vi "Auto Near Switch.vi"(9 "Time to wait (min 50ms)":dbl=50.0, 10 "Right?":bool) -> ()   [LabVIEW 2017]
uses:
  Auto switch direita.ctl
  LabVIEW_is_Under_Control.lib/Util/Unpack Gamepad/Button Cluster.ctl
  Team Code/Robot Global Data.vi
panel:
  in  "90_time_limit":dbl=1800.0
  in  "Time_limit_fwd_2":dbl=1500.0 format="%#_13g"
  in  "Time_Limit_fwd":dbl=4000.0 format="%#_13g"
  in  "Delay fwd 2":i32=10
  in  "DistanceAfterTurn":dbl=40.0
  in  "Delay Turn":i32=150
  in  "Turn":dbl=-90.0 format="%#_13g"
  in  "Delay Fwd":i32=100
  in  "DistanceSwitch":dbl=380.0
  out "auto state":T1=enum."Girando"
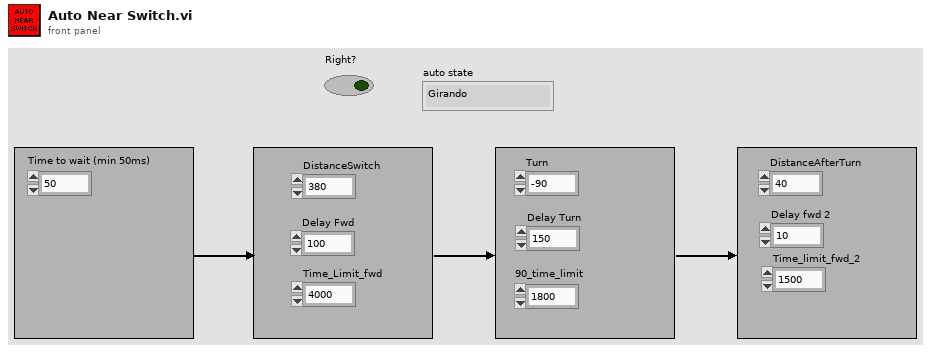
[diagram p1: front panel]
types:
  T1 = typedef "Auto switch direita.ctl" = enum16{"Zerandosensor", "Girando", "Andando", "Jogando", "Andando2", "Finalizando", "Zerandosensor2"}
  T2 = typedef "Button Cluster.ctl" = cluster{"Buttons[0]":bool, "Buttons[1]":bool, "Buttons[2]":bool, "Buttons[3]":bool, "Buttons[4]":bool, "Buttons[5]":bool, "Buttons[6]":bool, "Buttons[7]":bool, "Buttons[8]":bool, "Buttons[9]":bool}
  T3 = cluster{"proportional gain (Kc)":dbl, "integral time (Ti, min)":dbl, "derivative time (Td, min)":dbl}
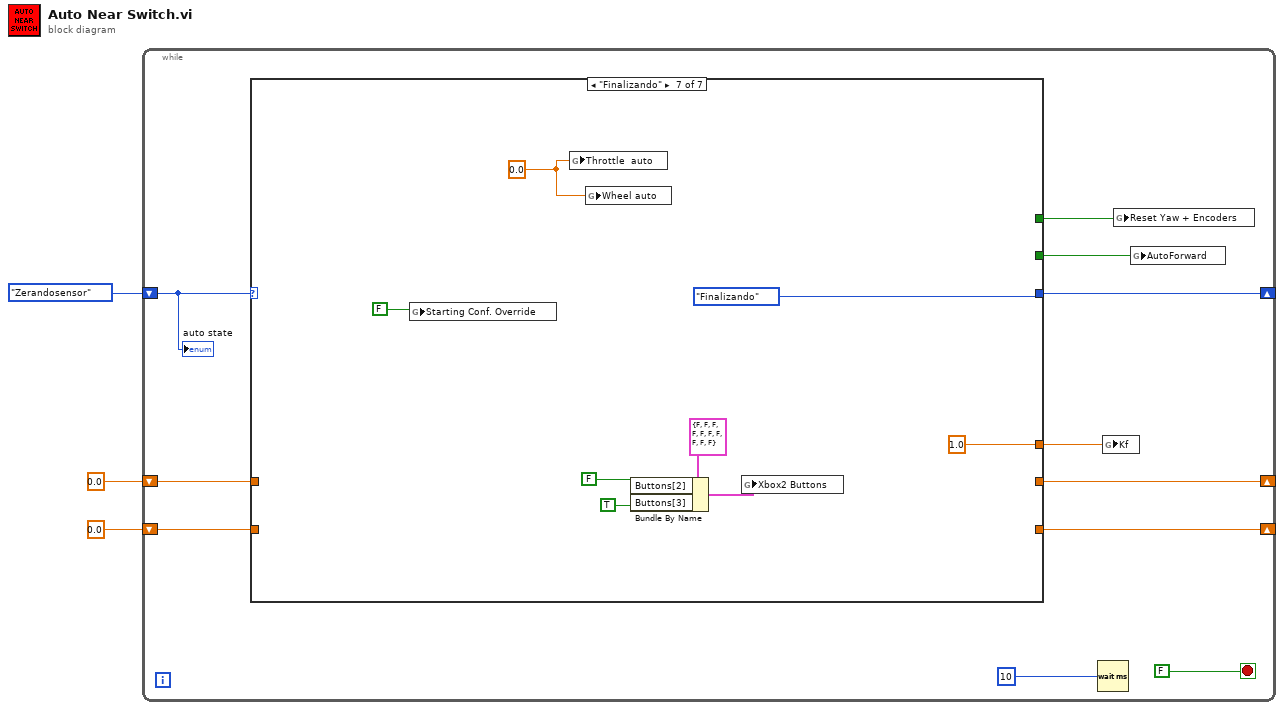
[diagram p0: block diagram]
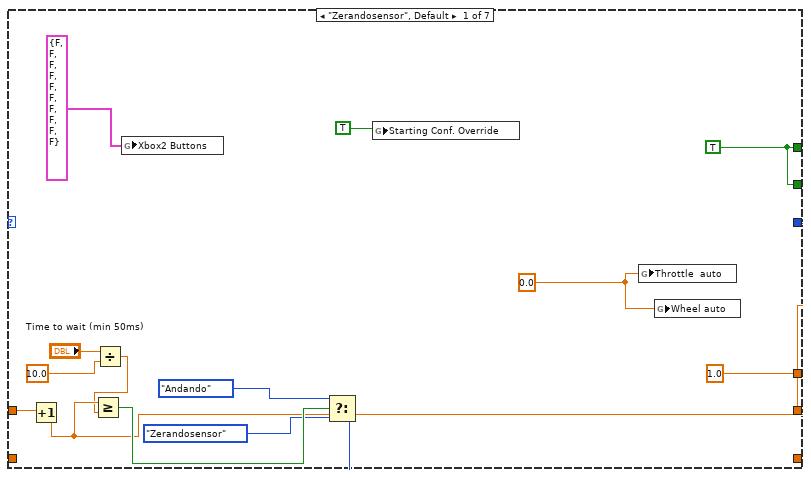
[diagram p2: hidden frame]
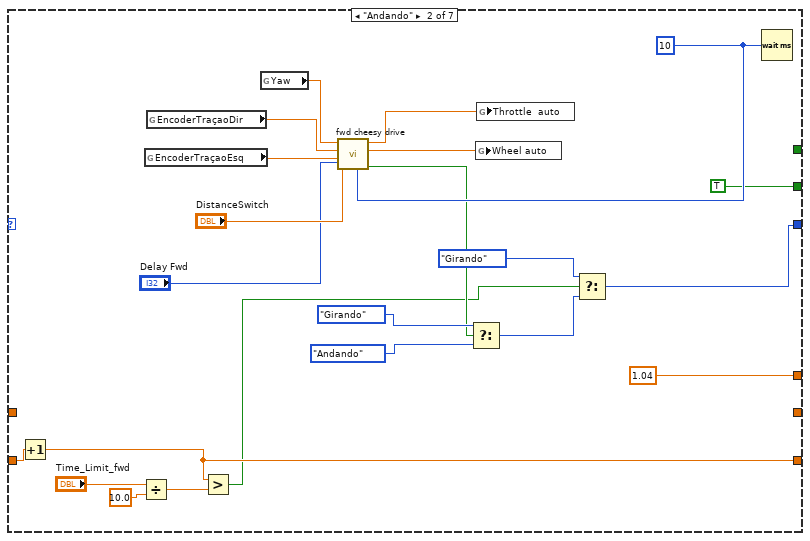
[diagram p3: hidden frame]
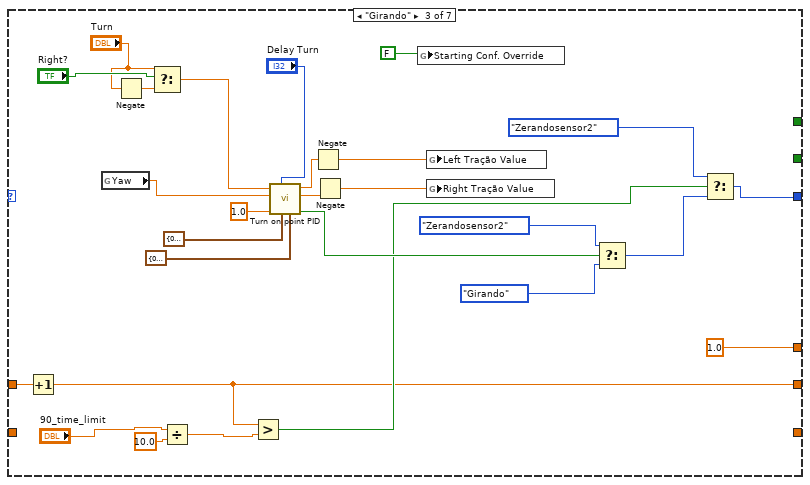
[diagram p4: hidden frame]
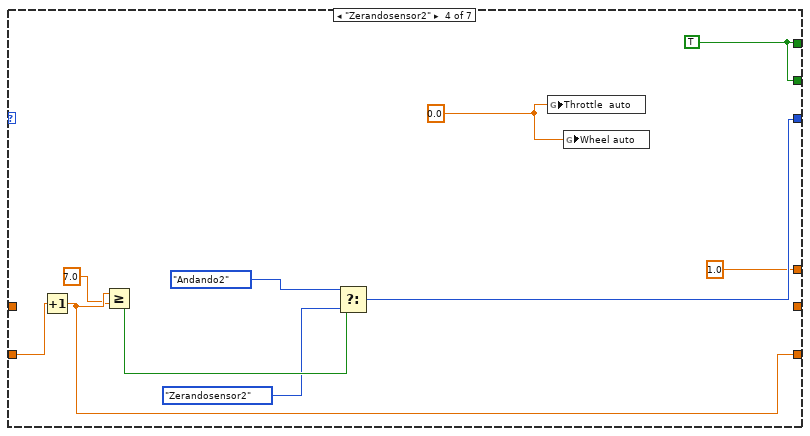
[diagram p5: hidden frame]
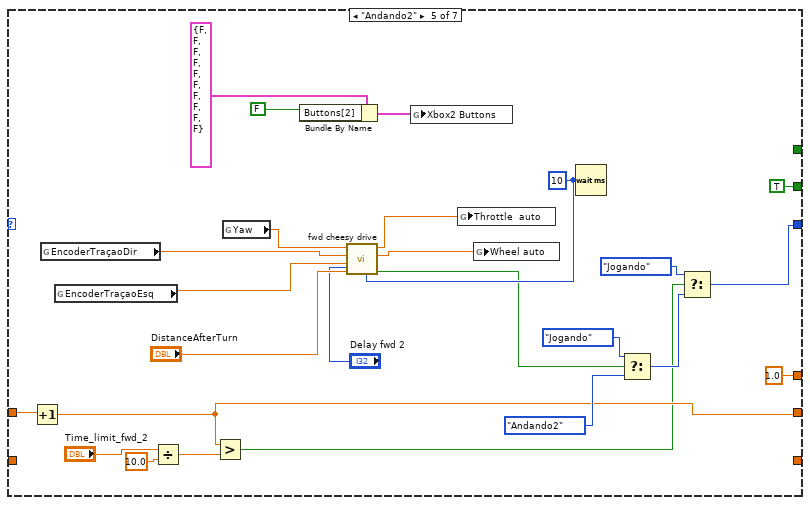
[diagram p6: hidden frame]
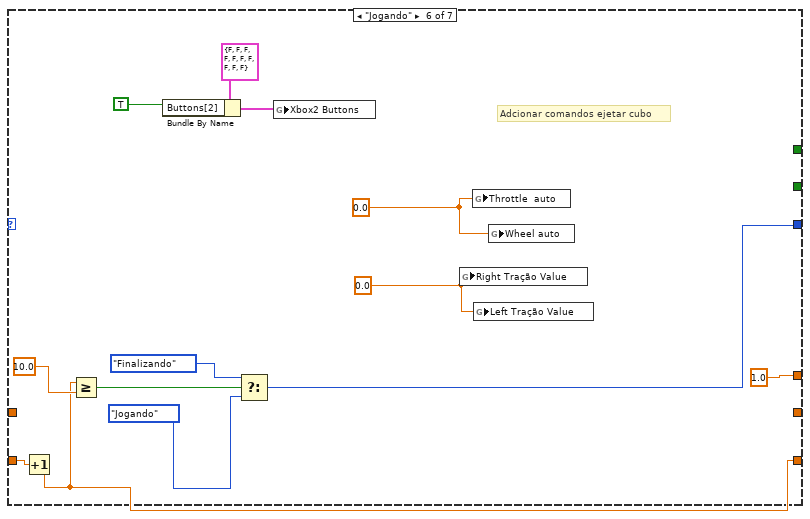
[diagram p7: hidden frame]
diagram:
  n1 = while {
    shift-right: [w10] -> _
    shift-left: Auto_switch_direita."Zerandosensor" -> [w8]
    shift-right: [w11] -> _
    shift-left: 0.0 -> [w12]
    shift-right: [w4] -> _
    shift-left: 0.0 -> [w5]
    stop <- FALSE stop-if-true
    n2 = case shown="\"Finalizando\"" w8 {
      tunnel: w12 -> [w19 _ w55 _ w98 _ _]
      tunnel: [w16 _ w54 _ w97 _ _] -> w11
      tunnel: [w27 w36 w57 w82 w93 w124 Auto_switch_direita."Finalizando"] -> w10
      tunnel: [w24 _ _ w86 _ _ _] -> w7
      tunnel: [w24 TRUE _ w86 TRUE _ _] -> w9
      tunnel: [1.0 1.04 1.0 1.0 1.0 1.0 1.0] -> w6
      tunnel: w5 -> [_ w32 _ w80 _ w120 _]
      tunnel: [_ w31 _ w79 _ w113 _] -> w4
      frame "Zerandosensor", Default {
        w23 = 0.0
        w24 = TRUE
        n3 = Increment(x=w19) -> (x+1=w16:dbl)
        n4 = Divide(x="Time to wait (min 50ms)", y=10.0) -> (x/y=w15:dbl)
        n5 = Greater Or Equal?(x=w16, y=w15) -> (x >= y?=w28:bool)
        n6 = global write "Robot Global Data.vi" "Xbox2 Buttons"(T2 {"Buttons[0]"=FALSE, "Buttons[1]"=FALSE, "Buttons[2]"=FALSE, "Buttons[3]"=FALSE, "Buttons[4]"=FALSE, "Buttons[5]"=FALSE, "Buttons[6]"=FALSE, "Buttons[7]"=FALSE, "Buttons[8]"=FALSE, "Buttons[9]"=FALSE} ("Madcatz Buttons")) -> ()
        n7 = Select(t=Auto_switch_direita."Andando", s=w28, f=Auto_switch_direita."Zerandosensor") -> (s? t:f=w27:T1)
        n8 = global write "Robot Global Data.vi" "Starting Conf. Override"(TRUE) -> ()
        n9 = global write "Robot Global Data.vi" "Throttle  auto"(w23) -> ()
        n10 = global write "Robot Global Data.vi" "Wheel auto"(w23) -> ()
      }
      frame "Andando" {
        w46 = u32 10 ("milliseconds to wait")
        n11 = Increment(x=w32) -> (x+1=w31:dbl)
        n12 = Divide(x="Time_Limit_fwd", y=10.0) -> (x/y=w33:dbl)
        n13 = global read "Robot Global Data.vi" "EncoderTraçaoEsq"() -> (w49:dbl)
        n14 = global read "Robot Global Data.vi" "EncoderTraçaoDir"() -> (w48:dbl)
        n15 = Greater?(x=w31, y=w33) -> (0:w29:bool)
        n16 = global read "Robot Global Data.vi" "Yaw"() -> (w50:dbl)
        n17 = call "fwd cheesy drive.vi"("Loop Timer"=w46, "Time to stop"="Delay Fwd", "Distance"="DistanceSwitch", "Encoder Left"=w49, "Encoder Right"=w48, "Yaw"=w50) -> ("Finished distance"=w30:bool, "Direction"=w44:dbl, "Trottle"=w43:dbl)  [unwired: 2 in, 1 out]
        n18 = Select(t=Auto_switch_direita."Girando", s=w30, f=Auto_switch_direita."Andando") -> (s? t:f=w37:T1)
        n19 = global write "Robot Global Data.vi" "Wheel auto"(w44) -> ()
        n20 = global write "Robot Global Data.vi" "Throttle  auto"(w43) -> ()
        n21 = Select(t=Auto_switch_direita."Girando", s=w29, f=w37) -> (s? t:f=w36:T1)
        n22 = Wait (ms)(milliseconds to wait=w46) -> ()  [unwired: 1 out]
      }
      frame "Girando" {
        n23 = Increment(x=w55) -> (x+1=w54:dbl)
        n24 = global read "Robot Global Data.vi" "Yaw"() -> (w70:dbl)
        n25 = Negate(x="Turn") -> (-x=w65:dbl)
        n26 = Select(t="Turn", s="Right?", f=w65) -> (s? t:f=w63:dbl)
        n27 = Divide(x="90_time_limit", y=10.0) -> (x/y=w61:dbl)
        n28 = Greater?(x=w54, y=w61) -> (0:w59:bool)
        n29 = call "Turn on point PID.vi"("Range"=cluster{"output high":dbl, "output low":dbl} {"output high"=0.65, "output low"=-0.65}, "Gains"=T3 {"proportional gain (Kc)"=0.015, "integral time (Ti, min)"=0.01, "derivative time (Td, min)"=0.0}, "Time to stop"="Delay Turn", "Precision"=1.0, "Yaw"=w70, "Setpoint(degrees)"=w63) -> ("Finished?"=w76:bool, "PWM right"=w72:dbl, "PWM left"=w73:dbl)  [unwired: 3 in]
        n30 = Negate(x=w73) -> (-x=w69:dbl)
        n31 = Negate(x=w72) -> (-x=w68:dbl)
        n32 = global write "Robot Global Data.vi" "Starting Conf. Override"(FALSE) -> ()
        n33 = global write "Robot Global Data.vi" "Left Tração Value"(w69) -> ()
        n34 = global write "Robot Global Data.vi" "Right Tração Value"(w68) -> ()
        n35 = Select(t=Auto_switch_direita."Zerandosensor2", s=w76, f=Auto_switch_direita."Girando") -> (s? t:f=w58:T1)
        n36 = Select(t=Auto_switch_direita."Zerandosensor2", s=w59, f=w58) -> (s? t:f=w57:T1)
      }
      frame "Zerandosensor2" {
        w86 = TRUE
        w87 = 0.0
        n37 = Increment(x=w80) -> (x+1=w79:dbl)
        n38 = Greater Or Equal?(x=w79, y=7.0) -> (x >= y?=w85:bool)
        n39 = Select(t=Auto_switch_direita."Andando2", s=w85, f=Auto_switch_direita."Zerandosensor2") -> (s? t:f=w82:T1)
        n40 = global write "Robot Global Data.vi" "Throttle  auto"(w87) -> ()
        n41 = global write "Robot Global Data.vi" "Wheel auto"(w87) -> ()
      }
      frame "Andando2" {
        w109 = u32 10 ("milliseconds to wait")
        n42 = Increment(x=w98) -> (x+1=w97:dbl)
        n43 = global read "Robot Global Data.vi" "EncoderTraçaoDir"() -> (w91:dbl)
        n44 = global read "Robot Global Data.vi" "EncoderTraçaoEsq"() -> (w111:dbl)
        n45 = Divide(x="Time_limit_fwd_2", y=10.0) -> (x/y=w99:dbl)
        n46 = Greater?(x=w97, y=w99) -> (0:w95:bool)
        n47 = global read "Robot Global Data.vi" "Yaw"() -> (w112:dbl)
        n48 = Bundle By Name(cluster=T2 {"Buttons[0]"=FALSE, "Buttons[1]"=FALSE, "Buttons[2]"=FALSE, "Buttons[3]"=FALSE, "Buttons[4]"=FALSE, "Buttons[5]"=FALSE, "Buttons[6]"=FALSE, "Buttons[7]"=FALSE, "Buttons[8]"=FALSE, "Buttons[9]"=FALSE} ("Xbox Buttons"), "Buttons[2]"=FALSE) -> (w89:T2)
        n49 = call "fwd cheesy drive.vi"("Loop Timer"=w109, "Time to stop"="Delay fwd 2", "Distance"="DistanceAfterTurn", "Encoder Left"=w111, "Encoder Right"=w91, "Yaw"=w112) -> ("Finished distance"=w92:bool, "Direction"=w107:dbl, "Trottle"=w106:dbl)  [unwired: 2 in, 1 out]
        n50 = global write "Robot Global Data.vi" "Xbox2 Buttons"(w89) -> ()
        n51 = global write "Robot Global Data.vi" "Throttle  auto"(w106) -> ()
        n52 = global write "Robot Global Data.vi" "Wheel auto"(w107) -> ()
        n53 = Wait (ms)(milliseconds to wait=w109) -> ()  [unwired: 1 out]
        n54 = Select(t=Auto_switch_direita."Jogando", s=w92, f=Auto_switch_direita."Andando2") -> (s? t:f=w96:T1)
        n55 = Select(t=Auto_switch_direita."Jogando", s=w95, f=w96) -> (s? t:f=w93:T1)
      }
      frame "Jogando" {
        w118 = 0.0
        w119 = 0.0
        # "Adcionar comandos ejetar cubo"
        n56 = Increment(x=w120) -> (x+1=w113:dbl)
        n57 = Greater Or Equal?(x=w113, y=10.0) -> (x >= y?=w125:bool)
        n58 = Bundle By Name(cluster=T2 {"Buttons[0]"=FALSE, "Buttons[1]"=FALSE, "Buttons[2]"=FALSE, "Buttons[3]"=FALSE, "Buttons[4]"=FALSE, "Buttons[5]"=FALSE, "Buttons[6]"=FALSE, "Buttons[7]"=FALSE, "Buttons[8]"=FALSE, "Buttons[9]"=FALSE} ("Xbox Buttons"), "Buttons[2]"=TRUE) -> (w116:T2)
        n59 = Select(t=Auto_switch_direita."Finalizando", s=w125, f=Auto_switch_direita."Jogando") -> (s? t:f=w124:T1)
        n60 = global write "Robot Global Data.vi" "Xbox2 Buttons"(w116) -> ()
        n61 = global write "Robot Global Data.vi" "Right Tração Value"(w118) -> ()
        n62 = global write "Robot Global Data.vi" "Throttle  auto"(w119) -> ()
        n63 = global write "Robot Global Data.vi" "Left Tração Value"(w118) -> ()
        n64 = global write "Robot Global Data.vi" "Wheel auto"(w119) -> ()
      }
      frame "Finalizando" {
        w131 = 0.0
        n65 = global write "Robot Global Data.vi" "Starting Conf. Override"(FALSE) -> ()
        n66 = global write "Robot Global Data.vi" "Throttle  auto"(w131) -> ()
        n67 = global write "Robot Global Data.vi" "Wheel auto"(w131) -> ()
        n68 = Bundle By Name(cluster=T2 {"Buttons[0]"=FALSE, "Buttons[1]"=FALSE, "Buttons[2]"=FALSE, "Buttons[3]"=FALSE, "Buttons[4]"=FALSE, "Buttons[5]"=FALSE, "Buttons[6]"=FALSE, "Buttons[7]"=FALSE, "Buttons[8]"=FALSE, "Buttons[9]"=FALSE} ("Xbox Buttons"), "Buttons[2]"=FALSE, "Buttons[3]"=TRUE) -> (w129:T2)
        n69 = global write "Robot Global Data.vi" "Xbox2 Buttons"(w129) -> ()
      }
    }
    n70 = Wait (ms)(milliseconds to wait=u32 10) -> ()  [unwired: 1 out]
    n71 = global write "Robot Global Data.vi" "Kf"(w6) -> ()
    n72 = global write "Robot Global Data.vi" "Reset Yaw + Encoders"(w7) -> ()
    n73 = global write "Robot Global Data.vi" "AutoForward"(w9) -> ()
    "auto state" <- w8
  }
